vi "citTemplate.Loop Example.vi"() -> ()   [LabVIEW 2019, in "Tools.lvlib"]
doc: "This is an example usage of CIT template."
uses:
  Tools.lvlib
  citTemplate.errData.ctl
panel:
  out "_loop":i32(ring)=4
types:
  T1 = typedef "Tools.lvlib/citTemplate.errData.ctl" = cluster{"action":string, "error":errorcluster}
  T2 = enum32{"idle", "constructor", "destructor", "--- Loop Name ---"}
  T3 = typedef "Tools.lvlib/citTemplate.notifierHandle.ctl" = refnum<notifier>
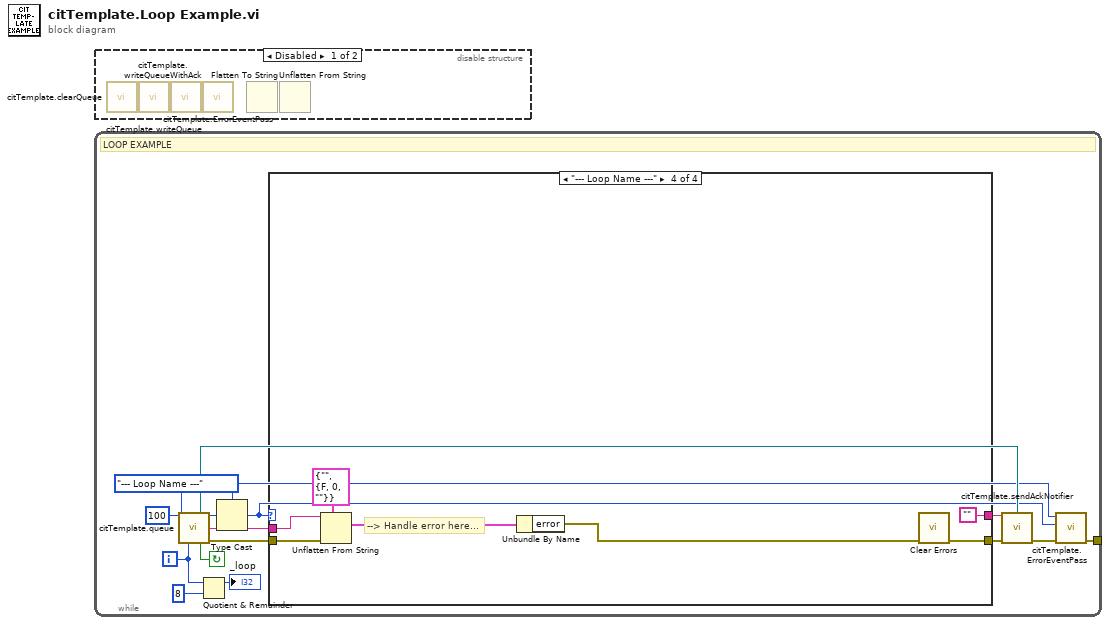
[diagram p0: block diagram]
diagram:
  n1 = while {
    tunnel: [w2] -> _
    i -> [w4]
    stop <- w11 continue-if-true
    w8 = T2."--- Loop Name ---" ("Action")
    # "LOOP EXAMPLE"
    n2 = call "citTemplate.queue.vi"("ms timeout (250 ms)"=100, "event enum"=w8, "iteration (-1)"=w4) -> ("notifierHandle out"=w10:T3, "event out"=w14:u32, "(flatten) data out"=w13:string, "continue"=w11:bool, "error out"=w12:errorcluster)  [unwired: 2 in, 6 out]
    n3 = Quotient & Remainder(x=w4, y=8) -> (x-y*floor(x/y)=→"_loop":i32)  [unwired: 1 out]
    n4 = Type Cast(type=w8, x=w14) -> (*(type *) &x=w3:T2)
    n5 = case shown="\"--- Loop Name ---\"" w3 {
      tunnel: w13 -> [_ _ _ w23]
      tunnel: w12 -> [w15 w16 w17 w21]
      tunnel: [_ _ _ ""] -> w9
      tunnel: [w15 w16 w17 w22] -> w7
      frame "idle" {
      }
      frame "constructor" {
      }
      frame "destructor" {
      }
      frame "--- Loop Name ---" {
        # "--> Handle error here..."
        n6 = Unflatten From String(type=T1 {"action"="", "error"={"status"=FALSE, "code"=0, "source"=""}} ("ErrData"), binary string=w23, error in (no error)=w21) -> (value=w19:T1)  [unwired: 4 out]
        n7 = Unbundle By Name(w19) -> ("error"=w18:errorcluster)
        n8 = call <vilib>:"Clear Errors.vi"("error in (no error)"=w18) -> ("error out"=w22:errorcluster)  [unwired: 5 in, 1 out]
      }
    }
    n9 = call "citTemplate.sendAckNotifier.vi"("notification data"=w9, "notifierHandle in"=w10, "error in"=w7) -> ()  [unwired: 13 out]
    n10 = call "citTemplate.ErrorEventPass.vi"("error in (no error)"=w7, "action of error"=w3, "event in"=w8) -> ("error out"=w2:errorcluster)  [unwired: 1 in, 7 out]
  }
  n11 = disable-structure shown="Disabled" {
    frame Disabled {
      n12 = call "citTemplate.clearQueue.vi"() -> ()  [unwired: 14 in, 2 out]
      n13 = call "citTemplate.writeQueue.vi"() -> ()  [unwired: 15 in, 1 out]
      n14 = call "citTemplate.writeQueueWithAck.vi"() -> ()  [unwired: 13 in, 3 out]
      n15 = call "citTemplate.ErrorEventPass.vi"() -> ()  [unwired: 11 in, 1 out]
      n16 = Flatten To String() -> ()  [unwired: 4 in, 3 out]
      n17 = Unflatten From String() -> ()  [unwired: 5 in, 3 out]
    }
    frame Enabled {
    }
  }
